vi "Get Server.vi"(11 "Processing in":refnum<class "Processing.lvclass">) -> (2 "Server":refnum<class "Server.lvclass">, 3 "Processing out":refnum<class "Processing.lvclass">)   [LabVIEW 2020, in "HTTP Server.lvlib" / "Processing.lvclass"]
uses:
  Processing.lvclass
  Processing.lvclass/Processing.ctl
  Server/Server.lvclass
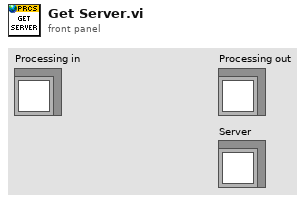
[diagram p1: front panel]
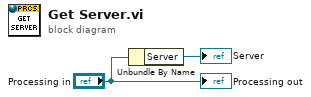
[diagram p0: block diagram]
diagram:
  n1 = Unbundle By Name("Processing in") -> ("Server"=→"Server":refnum<class "Server.lvclass">)
  "Processing out" <- "Processing in"
